vi "IMS Stepper Set Zero.vi"(1 "error in (no error)":errorcluster, 2 "Motor Number":u32=1 min=1 max=255 step=1, 3 "Instrument Address":refnum<visa-resource-name>) -> (0 "error out":errorcluster)   [LabVIEW 2018]
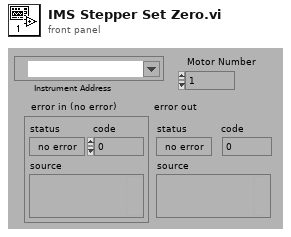
[diagram p1: front panel]
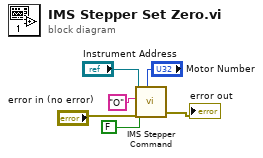
[diagram p0: block diagram]
diagram:
  n1 = call "IMS Stepper Command.vi"("Instrument Address"="Instrument Address", "Motor Number"="Motor Number", "Command"="O", "Mode"=FALSE, "error in (no error)"="error in (no error)") -> ("error out"=→"error out":errorcluster)  [unwired: 1 in, 2 out]
